vi "ResolutionEnumToRing.vi"(11 "resolution":T1) -> (3 "Resolutinon":u32(ring)=10 items=["1000 points"=1, "10k points"=10, "100k points"=100, "1M points"=1000, "5M points"=5000, "10M points"=10000])   [LabVIEW 2013, in "TektronixDPO.lvclass"]
uses:
  TektronixDPO.lvclass
  shared/Typdefs/Choice77.ctl
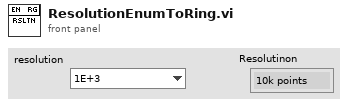
[diagram p1: front panel]
types:
  T1 = typedef "Choice77.ctl" = enum16{"1E+3", "10E+3", "100E+3", "1E+6", "5E+6", "10E+6"}
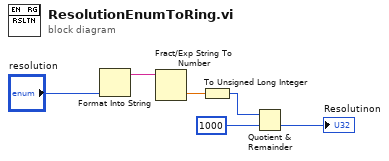
[diagram p0: block diagram]
diagram:
  n1 = Format Into String("resolution") -> (resulting string=w3:string)  [unwired: 3 in, 1 out]
  n2 = Fract/Exp String To Number(string=w3) -> (number=w4:dbl)  [unwired: 3 in, 1 out]
  n3 = To Unsigned Long Integer(number=w4) -> (unsigned 32bit integer=w5:u32)
  n4 = Quotient & Remainder(x=w5, y=u32 1000) -> (floor(x/y)=→"Resolutinon":u32)  [unwired: 1 out]
